vi "line to strings.vi"(11 "line":T1={"ID"="", "Setpoint"=refnum, "Process Variable"=refnum, "Output"=refnum, "PID gains"={"proportional gain (Kc)"=1.0, "integral time (Ti, min)"=0.01, "derivative time (Td, min)"=0.0}, "output range"={"output high"=100.0, "output low"=-100.0}} {"output range"."output low" format="%.2f"; "output range"."output high" format="%.2f"; "PID gains"."proportional gain (Kc)" format="%.2f"; "PID gains"."integral time (Ti, min)" format="%.2f"}) -> (3 "strings":string[](array[string]))   [LabVIEW 2014, in "Tagbus PID Module editor node.lvclass"]
uses:
  Tagbus PID Module editor node.lvclass
  table line.ctl
  <vilib>/NI/Tag Bus Module Framework/channel/TBM channel.lvclass
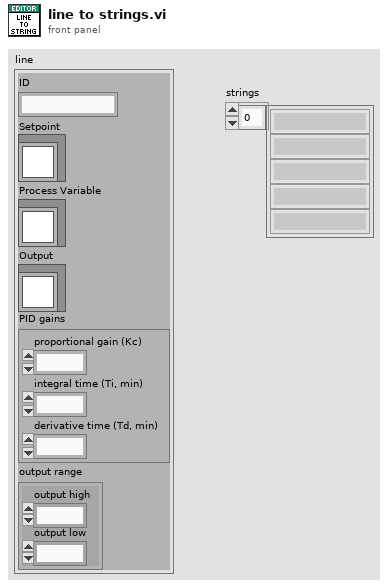
[diagram p1: front panel]
types:
  T1 = typedef "Tagbus PID Module editor node.lvclass/table line.ctl" = cluster{"ID":string, "Setpoint":refnum<class "TBM channel.lvclass">, "Process Variable":refnum<class "TBM channel.lvclass">, "Output":refnum<class "TBM channel.lvclass">, "PID gains":cluster{"proportional gain (Kc)":dbl, "integral time (Ti, min)":dbl, "derivative time (Td, min)":dbl}, "output range":cluster{"output high":dbl, "output low":dbl}}
  T2 = cluster{"proportional gain (Kc)":dbl, "integral time (Ti, min)":dbl, "derivative time (Td, min)":dbl}
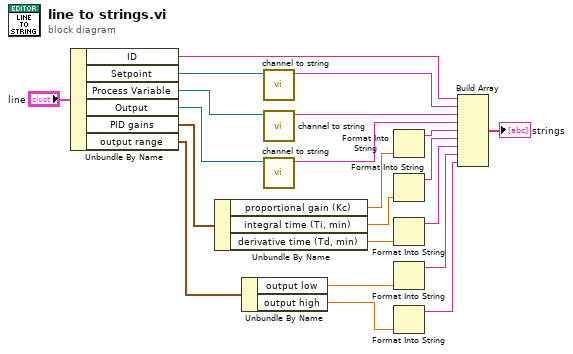
[diagram p0: block diagram]
diagram:
  n1 = Unbundle By Name("line") -> ("ID"=w20:string, "Setpoint"=w6:refnum<class "TBM channel.lvclass">, "Process Variable"=w4:refnum<class "TBM channel.lvclass">, "Output"=w3:refnum<class "TBM channel.lvclass">, "PID gains"=w18:T2, "output range"=w11:cluster{"output high":dbl, "output low":dbl})
  n2 = Unbundle By Name(w18) -> ("proportional gain (Kc)"=w17:dbl, "integral time (Ti, min)"=w16:dbl, "derivative time (Td, min)"=w15:dbl)
  n3 = Unbundle By Name(w11) -> ("output low"=w10:dbl, "output high"=w9:dbl)
  n4 = call <vilib>:"channel to string.vi"("channel in"=w6) -> ("identifier"=w5:string)  [unwired: 9 in, 1 out]
  n5 = call <vilib>:"channel to string.vi"("channel in"=w4) -> ("identifier"=w2:string)  [unwired: 9 in, 1 out]
  n6 = call <vilib>:"channel to string.vi"("channel in"=w3) -> ("identifier"=w1:string)  [unwired: 9 in, 1 out]
  n7 = Format Into String(w17) -> (resulting string=w14:string)  [unwired: 3 in, 1 out]
  n8 = Format Into String(w16) -> (resulting string=w13:string)  [unwired: 3 in, 1 out]
  n9 = Format Into String(w15) -> (resulting string=w12:string)  [unwired: 3 in, 1 out]
  n10 = Format Into String(w10) -> (resulting string=w8:string)  [unwired: 3 in, 1 out]
  n11 = Format Into String(w9) -> (resulting string=w7:string)  [unwired: 3 in, 1 out]
  n12 = Build Array(w20, w5, w2, w1, w14, w13, w12, w8, w7) -> (→"strings":string[])
